vi "Parallel DAQ Events.vi"() -> ()   [LabVIEW 2020]
panel:
  in  "Event Based":bool
  out "Chart":waveform(dbl)[](graph)
  in  "stop":bool
  # "This example demonstrates running enough parallel DAQmx tasks to potentially cause issues with the LV execution system.\n\nBefore running this VI, set the \"Event Based\" boolean to the value you'd like to run at and see the differences in behavior.\n\nNote: It is expected to periodically see a chunk of missing data  in the chart. This is an artifact of the simplistic collation implementation that collects data from the parallel tasks tp generate the chart data and isn't a problem with the DAQmx data collection itself.\n\nThe key takeaway here is that enabling the event based acquisition should show a consistent separation between the data collected from tasks.\n\nWhen disabling the event based acquisition you should see that the data from the later tasks is spread out more and everytime this VI is run there will be variable start timing for those later tasks.\n\nAdditional comments are on the block diagram to describe more details about the implementation."
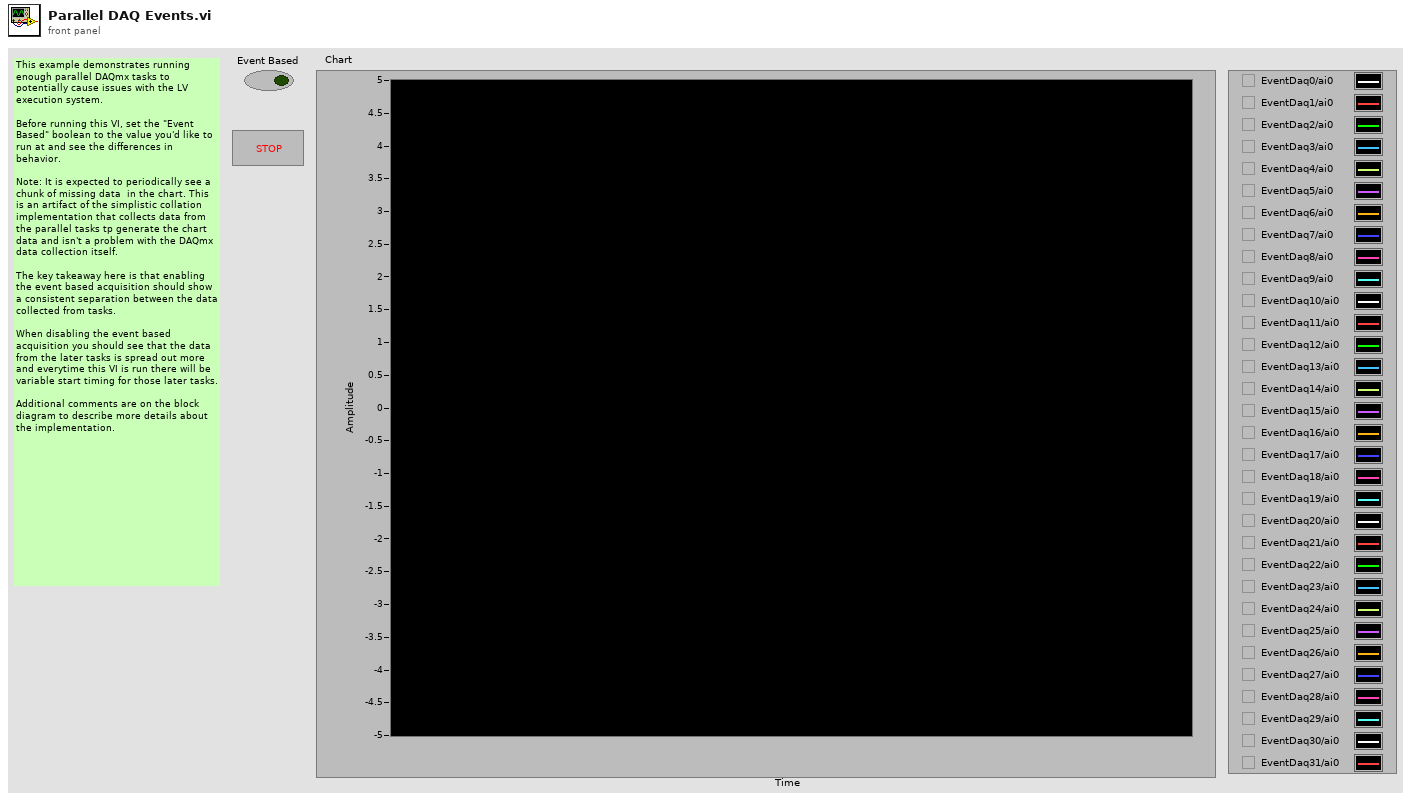
[diagram p1: front panel]
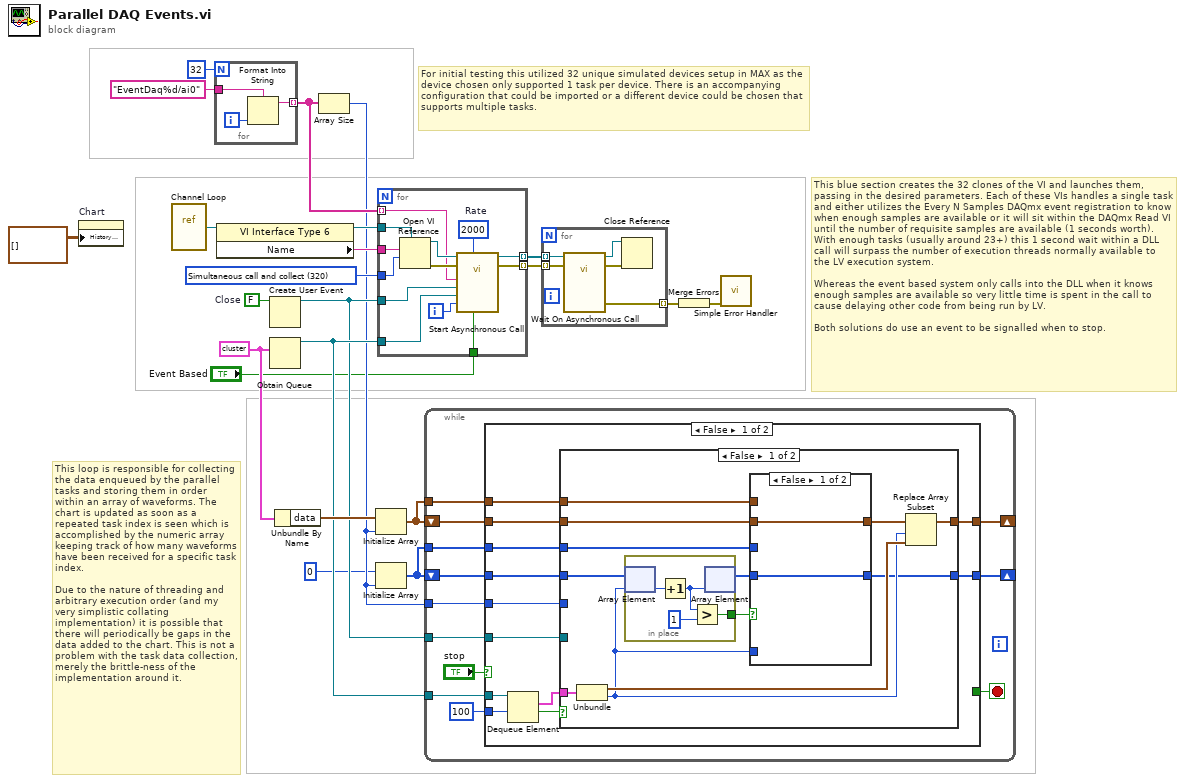
[diagram p0: block diagram]
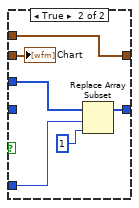
[diagram p2: hidden frame]
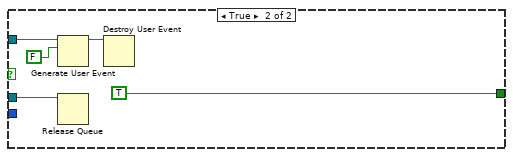
[diagram p4: hidden frame]
diagram:
  w17 = cluster{"data":waveform(dbl), "Index":i32} {"data"={"t0"=timestamp(0 s since 1904-01-01), "dt"=0.0, "Y"=[]}, "Index"=0}
  w18 = FALSE  # Close
  w19 = 320 items=["Record modifications"=1, "Open templates for editing"=2, "Prompt user to save"=4, "Prepare for reentrant run"=8, "Prompt to find missing subVIs"=16, "Hide loading dialog box"=32, "Enable simultaneous calls"=64, "Prepare to call and forget"=128, "Simultaneous call and forget"=192, "Prepare to call and collect"=256, "Simultaneous call and collect"=320]
  # "This loop is responsible for collecting the data enqueued by the parallel tasks and storing them in order within an array of waveforms. The chart is updated as soon as a repeated task index is seen which is accomplished by the numeric array keeping track of how many waveforms have been received for a specific task index.\n\nDue to the nature of threading and arbitrary execution order (and my very simplistic collating implementation) it is possible that there will periodically be gaps in the data added to the chart. This is not a problem with the task data collection, merely the brittle-ness of the implementation around it."
  # "This blue section creates the 32 clones of the VI and launches them, passing in the desired parameters. Each of these VIs handles a single task and either utilizes the Every N Samples DAQmx event registration to know when enough samples are available or it will sit within the DAQmx Read VI until the number of requisite samples are available (1 seconds worth). With enough tasks (usually around 23+) this 1 second wait within a DLL call will surpass the number of execution threads normally available to the LV execution system.\n\nWhereas the event based system only calls into the DLL when it knows enough samples are available so very little time is spent in the call to cause delaying other code from being run by LV.\n\nBoth solutions do use an event to be signalled when to stop."
  # "For initial testing this utilized 32 unique simulated devices setup in MAX as the device chosen only supported 1 task per device. There is an accompanying configuration that could be imported or a different device could be chosen that supports multiple tasks."
  n1 = property on="Chart" class="WFChart (strict)"("History Data"=waveform(dbl)[][] []) -> ()  [unwired: 2 in, 2 out]
  n2 = vi-ref "Channel Loop.vi"() -> (w22:refnum<vi>)
  n3 = for {
    N: 32 -> [_]
    tunnel: "EventDaq%d/ai0" -> [w24]
    tunnel: [w25] -> w8 mode=indexing
    i -> [w23]
    n4 = Format Into String(format string=w24, w23) -> (resulting string=w25:string)  [unwired: 2 in, 1 out]
  }
  n5 = property class="VI Interface Type 6"(reference=w22) -> (reference out=w21:refnum<vi>, "Name"=w20:string)  [unwired: 1 in, 1 out]
  n6 = Create User Event(user event datatype=w18) -> (user event=w13:refnum<user-event>)  [unwired: 1 in, 1 out]
  n7 = Obtain Queue(element data type=w17) -> (queue out=w14:refnum<queue>)  [unwired: 4 in, 2 out]
  n8 = Unbundle By Name(w17) -> ("data"=w16:waveform(dbl))
  n9 = Array Size(array=w8) -> (size(s)=w7:i32)
  n10 = Initialize Array(w16, w7) -> (w15:waveform(dbl)[])
  n11 = Initialize Array(0, w7) -> (w5:i32[])
  n12 = for {
    tunnel: w8 -> [w33] mode=indexing
    tunnel: w21 -> [w36]
    tunnel: w20 -> [w35]
    tunnel: w19 -> [w34]
    tunnel: w13 -> [w32]
    tunnel: w14 -> [w31]
    tunnel: [w29] -> w11 mode=indexing
    tunnel: [w28] -> w12 mode=indexing
    tunnel: "Event Based" -> [w26]
    i -> [w30]
    w27 = 2000  # Rate
    n13 = Open VI Reference(type specifier VI Refnum (for type only)=w36, vi path=w35, options=w34) -> (vi reference=w37:refnum<vi>, error out=w38:errorcluster)  [unwired: 3 in]
    n14 = call-by-ref "Start Asynchronous Call"(reference=w37, error in=w38, "Event Based?"=w26, "Rate"=w27, "Index"=w30, "Waveform Queue"=w31, "Close Event"=w32, "Channel"=w33) -> (reference out=w28:refnum<vi>, error out=w29:errorcluster)  [unwired: 5 in, 1 out]
  }
  n15 = while {
    shift-right: [w48] -> _
    shift-left: w15 -> [w49]
    tunnel: w15 -> [w47]
    tunnel: w14 -> [w50]
    tunnel: w13 -> [w46]
    shift-right: [w43] -> _
    shift-left: w5 -> [w44]
    tunnel: w7 -> [w42]
    tunnel: w5 -> [w41]
    stop <- w45 stop-if-true
    n16 = case shown="False" "stop" {
      tunnel: w50 -> [w62 w90]
      tunnel: w49 -> [w59 _]
      tunnel: [w58 _] -> w48
      tunnel: w47 -> [w57 _]
      tunnel: w46 -> [w56 w91]
      tunnel: [_ TRUE] -> w45
      tunnel: w44 -> [w55 _]
      tunnel: [w54 _] -> w43
      tunnel: w42 -> [w53 _]
      tunnel: w41 -> [w52 _]
      tunnel: 100 ("t") -> [w51 _]
      frame False {
        n17 = Dequeue Element(queue=w62, timeout in ms (-1)=w51) -> (element=w60:cluster{"data":waveform(dbl), "Index":i32}, timed out?=w61:bool)  [unwired: 1 in, 2 out]
        n18 = case shown="False" w61 {
          tunnel: w60 -> [w74 _]
          tunnel: w59 -> [w66 w88]
          tunnel: [w63 w88] -> w58
          tunnel: w57 -> [w72 _]
          tunnel: w56 -> [_ _]
          tunnel: w55 -> [w71 w87]
          tunnel: [w65 w87] -> w54
          tunnel: w53 -> [_ _]
          tunnel: w52 -> [w68 _]
          frame False {
            n19 = Unbundle(w74) -> ("data"=w73:waveform(dbl), "Index"=w67:i32)
            n20 = in-place {
              in-place-border: [w75] -> w70
              n21 = in-place-array #1(w71, w67) -> (w78:i32)
              n22 = Increment(x=w78) -> (x+1=w76:i32)
              n23 = Greater?(x=w76, y=1) -> (0:w75:bool)
              n24 = in-place-array #1(w76) -> (w69:i32[])  [unwired: 1 out]
            }
            n25 = case shown="False" w70 {
              tunnel: w72 -> [_ w86]
              tunnel: [w80 w86] -> w64
              tunnel: w66 -> [w80 w85]
              tunnel: w69 -> [w79 _]
              tunnel: w68 -> [_ w84]
              tunnel: w67 -> [_ w83]
              tunnel: [w79 w81] -> w65
              frame False {
              }
              frame True {
                n26 = Replace Array Subset(array=w84, new element=1 ("new element/subarray"), index=w83) -> (w81:i32[])
                "Chart" <- w85
              }
            }
            n27 = Replace Array Subset(array=w64, new element=w73, index=w67) -> (w63:waveform(dbl)[])
          }
          frame True {
          }
        }
      }
      frame True {
        n28 = Generate User Event(user event=w91, event data cluster=FALSE) -> (user event out=w93:refnum<user-event>)  [unwired: 2 in, 1 out]
        n29 = Release Queue(queue=w90) -> ()  [unwired: 2 in, 3 out]
        n30 = Destroy User Event(user event=w93) -> ()  [unwired: 1 in, 1 out]
      }
    }
  }
  n31 = for {
    tunnel: w12 -> [w98] mode=indexing
    tunnel: w11 -> [w97] mode=indexing
    tunnel: [w96] -> w2 mode=indexing
    n32 = call-by-ref "Wait On Asynchronous Call"(reference=w98, error in=w97) -> (reference out=w94:refnum<vi>, error out=w95:errorcluster, 0:"error out"=w96:errorcluster)  [unwired: 11 in]
    n33 = Close Reference(reference=w94, error in (no error)=w95) -> ()  [unwired: 1 out]
  }
  n34 = Merge Errors(w2) -> (w1:errorcluster)
  n35 = call <vilib>:"Simple Error Handler.vi"("error in (no error)"=w1) -> ()  [unwired: 4 in, 5 out]
